vi "ReadandMedianSR830_ETH_copy2.vi"(0 "data storage rate (Hz)":u16(ring)=7 items=[".0625 ", "0.125 ", "0.250 ", "0.500 ", "1 ", "2 ", "4", "8 ", "16 ", "32 ", "64 ", "128", "256", "512"], 1 "Lockin Address":string="0:8", 2 "Integration (ms)":u32=10000, 3 "Delay (ms)":u32=3000, 4 "Measure Mode\n(T =Signal)":bool=TRUE, 5 "error in":T1) -> (6 "signal (complex)":cdb, 7 "Frequency (Hz)":dbl, 8 "error out":T1)   [LabVIEW 2023]
uses:
  <vilib>/Analysis/NI_AALBase.lvlib
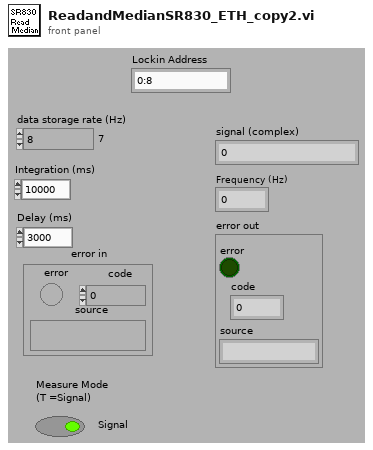
[diagram p1: front panel]
types:
  T1 = cluster{"error":bool, "code":i32, "source":string}
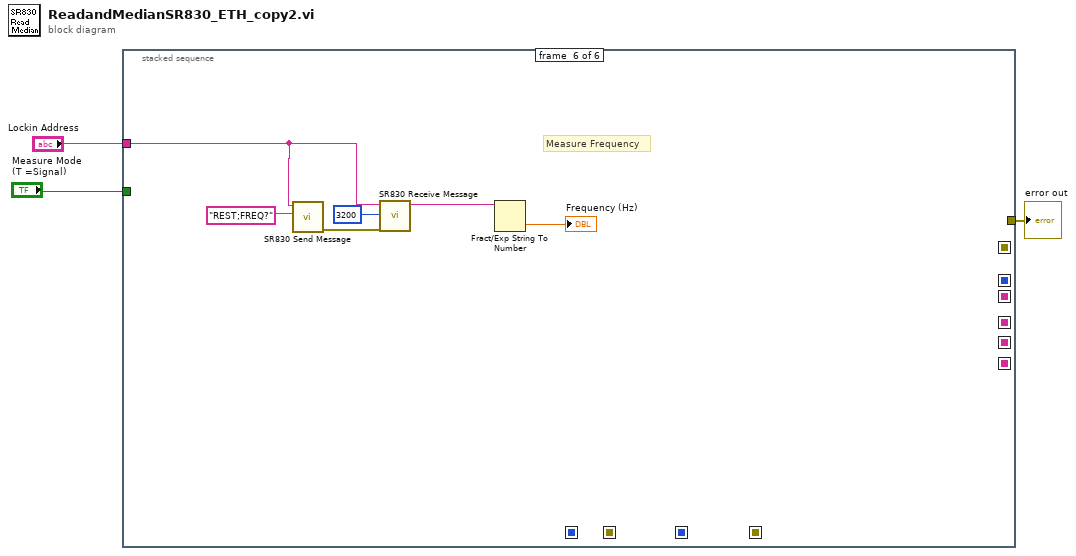
[diagram p0: block diagram]
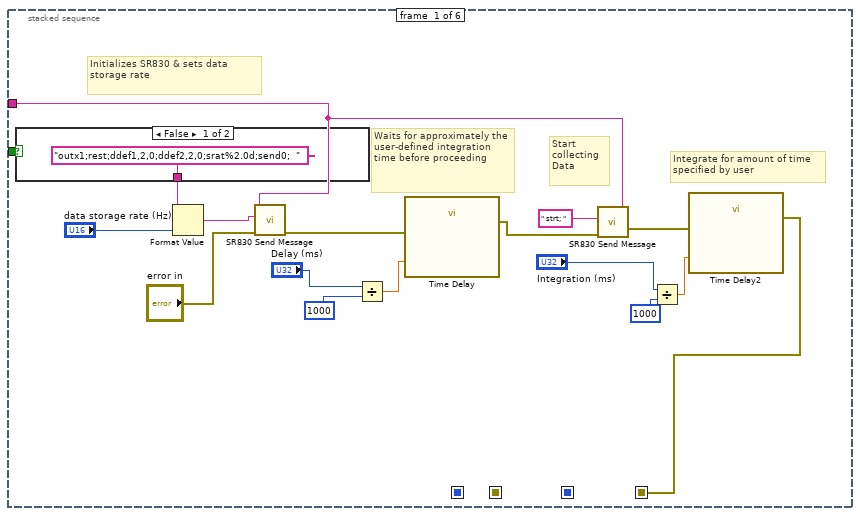
[diagram p2: hidden frame]
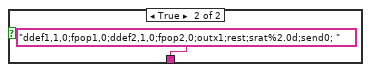
[diagram p3: hidden frame]
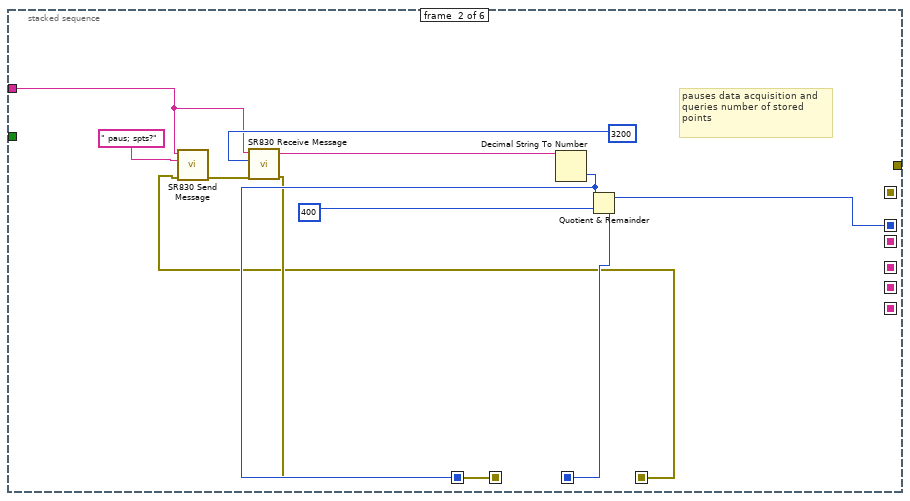
[diagram p4: hidden frame]
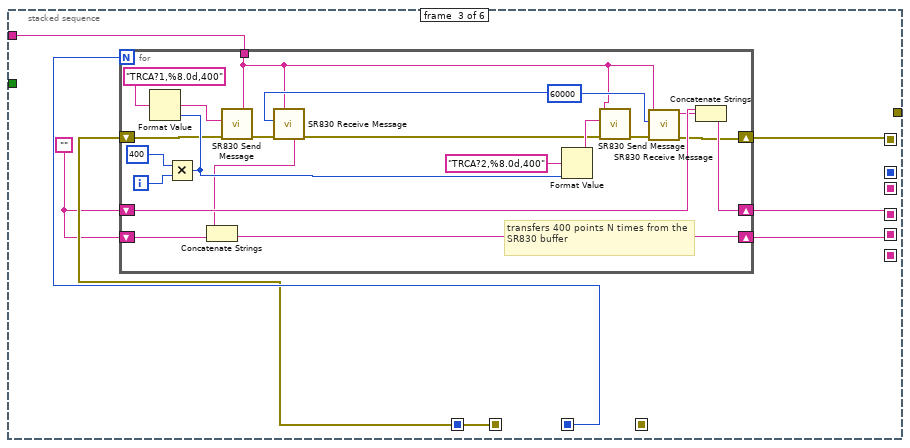
[diagram p5: hidden frame]
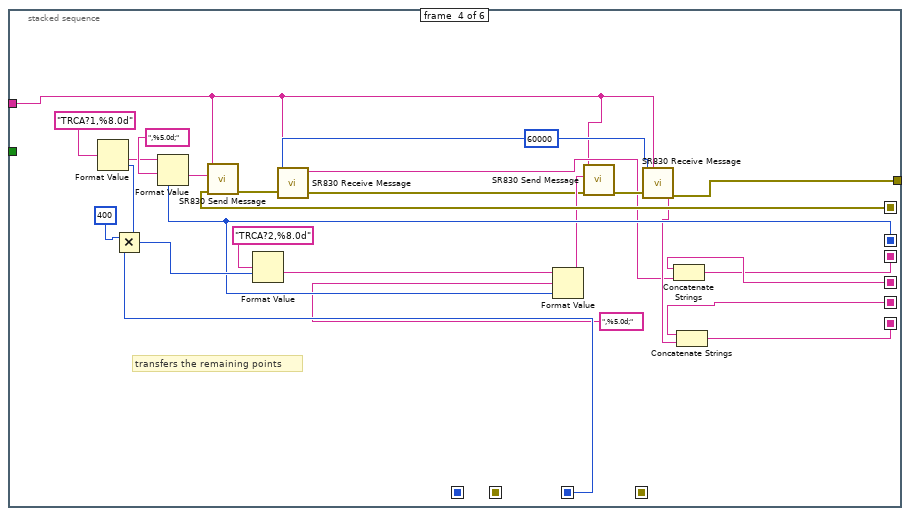
[diagram p6: hidden frame]
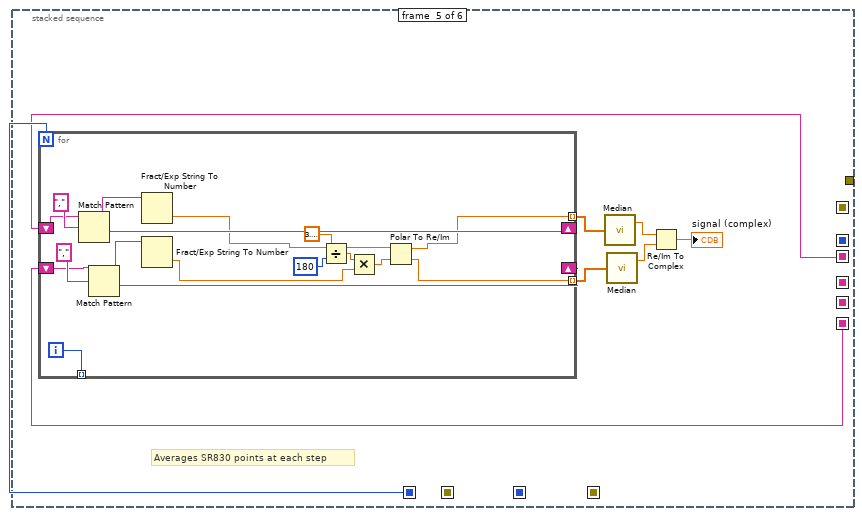
[diagram p7: hidden frame]
diagram:
  n1 = stacked-sequence {
    seq-local: [_ w32 _ _ _ _] -> [_ _ _ w82 _ _]
    seq-local: [_ w31 _ _ _ _] -> [_ _ w40 w84 _ _]
    seq-local: [_ w25 _ _ _ _] -> [_ _ w39 _ _ _]
    seq-local: [_ _ w37 _ _ _] -> [_ _ _ w79 _ _]
    seq-local: [_ _ w36 _ _ _] -> [_ _ _ w81 _ _]
    seq-local: [_ _ w35 _ _ _] -> [_ _ _ w80 _ _]
    seq-local: [_ w30 _ _ _ _] -> [_ _ _ _ w93 _]
    seq-local: [_ _ _ w64 _ _] -> [_ _ _ _ w91 _]
    seq-local: [_ _ _ w63 _ _] -> [_ _ _ _ w92 _]
    seq-local: [w17 _ _ _ _ _] -> [_ w24 _ _ _ _]
    tunnel: [_ _ _ w62 _ _] -> w3
    tunnel: "Lockin Address" -> [w5 w23 w34 w61 _ w116]
    tunnel: "Measure Mode\n(T =Signal)" -> [w4 _ _ _ _ _]
    frame #0 {
      # "Initializes SR830 & sets data storage rate"
      # "Integrate for amount of time\nspecified by user"
      # "Waits for approximately the user-defined integration time before proceeding"
      # "Start collecting Data"
      n2 = case shown="False" w4 {
        tunnel: ["outx1;rest;ddef1,2,0;ddef2,2,0;srat%2.0d;send0;  " "ddef1,1,0;fpop1,0;ddef2,1,0;fpop2,0;outx1;rest;srat%2.0d;send0; "] -> w15
        frame False {
        }
        frame True {
        }
      }
      n3 = Format Value(format string=w15, value (0)="data storage rate (Hz)") -> (output string=w13:string)  [unwired: 1 in]
      n4 = call "SR830 Send Message.vi"("address string"=w5, "write buffer"=w13, "error in"="error in") -> ("error out"=w16:T1)  [unwired: 4 in, 2 out]
      n5 = Divide(x="Delay (ms)", y=1000) -> (x/y=w9:dbl)
      n6 = call "Time Delay"("error in (no error)"=w16, "Delay Time (s)"=w9) -> ("error out"=w19:errorcluster)  [unwired: 9 in]
      n7 = call "SR830 Send Message.vi"("address string"=w5, "write buffer"=" strt; ", "error in"=w19) -> ("error out"=w18:T1)  [unwired: 4 in, 2 out]
      n8 = Divide(x="Integration (ms)", y=1000) -> (x/y=w6:dbl)
      n9 = call "Time Delay2"("error in (no error)"=w18, "Delay Time (s)"=w6) -> ("error out"=w17:errorcluster)  [unwired: 9 in]
    }
    frame #1 {
      # "pauses data acquisition and queries number of stored points"
      n10 = call "SR830 Send Message.vi"("address string"=w23, "write buffer"=" paus; spts?", "error in"=w24) -> ("error out"=w28:T1)  [unwired: 4 in, 2 out]
      n11 = call "SR830 Receive Message.vi"("address string"=w23, "byte count"=3200, "error in"=w28) -> ("read buffer"=w26:string, "error out"=w25:T1)  [unwired: 4 in, 1 out]
      n12 = Decimal String To Number(string=w26) -> (number=w30:i32)  [unwired: 2 in, 1 out]
      n13 = Quotient & Remainder(x=w30, y=400) -> (x-y*floor(x/y)=w32:i32, floor(x/y)=w31:i32)
    }
    frame #2 {
      w38 = ""
      n14 = for {
        N: w40 -> [_]
        shift-right: [w46] -> w37
        shift-left: w39 -> [w53]
        shift-right: [w58] -> w35
        shift-left: w38 -> [w57]
        shift-right: [w54] -> w36
        shift-left: w38 -> [w55]
        tunnel: w34 -> [w41]
        i -> [w60]
        w47 = 60000
        # "transfers 400 points N times from the SR830 buffer"
        n15 = Multiply(x=400, y=w60) -> (x*y=w56:i32)
        n16 = Format Value(format string="TRCA?1,%8.0d,400", value (0)=w56) -> (output string=w51:string)  [unwired: 1 in]
        n17 = call "SR830 Send Message.vi"("address string"=w41, "write buffer"=w51, "error in"=w53) -> ("error out"=w52:T1)  [unwired: 4 in, 2 out]
        n18 = call "SR830 Receive Message.vi"("address string"=w41, "byte count"=w47, "error in"=w52) -> ("read buffer"=w50:string, "error out"=w48:T1)  [unwired: 4 in, 1 out]
        n19 = Concatenate Strings(w50, w57) -> (w58:string)
        n20 = Format Value(format string="TRCA?2,%8.0d,400", value (0)=w56) -> (output string=w49:string)  [unwired: 1 in]
        n21 = call "SR830 Send Message.vi"("address string"=w41, "write buffer"=w49, "error in"=w48) -> ("error out"=w45:T1)  [unwired: 4 in, 2 out]
        n22 = call "SR830 Receive Message.vi"("address string"=w41, "byte count"=w47, "error in"=w45) -> ("read buffer"=w44:string, "error out"=w46:T1)  [unwired: 4 in, 1 out]
        n23 = Concatenate Strings(w55, w44) -> (w54:string)
      }
    }
    frame #3 {
      w73 = 60000
      # "transfers the remaining points"
      n24 = Multiply(x=400, y=w84) -> (x*y=w83:i32)
      n25 = Format Value(format string="TRCA?1,%8.0d", value (0)=w83) -> (output string=w69:string)  [unwired: 1 in]
      n26 = Format Value(string ("")=w69, format string=",%5.0d;", value (0)=w82) -> (output string=w68:string)
      n27 = call "SR830 Send Message.vi"("address string"=w61, "write buffer"=w68, "error in"=w79) -> ("error out"=w75:T1)  [unwired: 4 in, 2 out]
      n28 = Format Value(format string="TRCA?2,%8.0d", value (0)=w83) -> (output string=w65:string)  [unwired: 1 in]
      n29 = call "SR830 Receive Message.vi"("address string"=w61, "byte count"=w73, "error in"=w75) -> ("read buffer"=w74:string, "error out"=w72:T1)  [unwired: 4 in, 1 out]
      n30 = Format Value(string ("")=w65, format string=",%5.0d;", value (0)=w82) -> (output string=w78:string)
      n31 = call "SR830 Send Message.vi"("address string"=w61, "write buffer"=w78, "error in"=w72) -> ("error out"=w77:T1)  [unwired: 4 in, 2 out]
      n32 = call "SR830 Receive Message.vi"("address string"=w61, "byte count"=w73, "error in"=w77) -> ("read buffer"=w76:string, "error out"=w62:T1)  [unwired: 4 in, 1 out]
      n33 = Concatenate Strings(w81, w74) -> (w64:string)
      n34 = Concatenate Strings(w80, w76) -> (w63:string)
    }
    frame #4 {
      # "Averages SR830 points at each step"
      n35 = for {
        N: w93 -> [_]
        shift-right: [w106] -> _
        shift-left: w91 -> [w105]
        shift-right: [w104] -> _
        shift-left: w92 -> [w103]
        tunnel: [w102] -> _ mode=indexing
        tunnel: [w99] -> w89 mode=indexing
        tunnel: [w98] -> w88 mode=indexing
        i -> [w102]
        n36 = Match Pattern(string=w105, regular expression=",") -> (before substring=w109:string, after substring=w106:string)  [unwired: 1 in, 2 out]
        n37 = Match Pattern(string=w103, regular expression=",") -> (before substring=w108:string, after substring=w104:string)  [unwired: 1 in, 2 out]
        n38 = Fract/Exp String To Number(string=w109) -> (number=w100:dbl)  [unwired: 3 in, 1 out]
        n39 = Fract/Exp String To Number(string=w108) -> (number=w101:dbl)  [unwired: 3 in, 1 out]
        n40 = Divide(x=3.141592653589793, y=180) -> (x/y=w95:dbl)
        n41 = Multiply(x=w95, y=w101) -> (x*y=w94:dbl)
        n42 = Polar To Re/Im(2:w94, 3:w100) -> (0:w98:dbl, 1:w99:dbl)
      }
      n43 = call <vilib>:"Median.vi"("X"=w89) -> ("median"=w86:dbl)  [unwired: 1 out]
      n44 = call <vilib>:"Median.vi"("X"=w88) -> ("median"=w87:dbl)  [unwired: 1 out]
      n45 = Re/Im To Complex(1:w87, 2:w86) -> (0:→"signal (complex)":cdb)
    }
    frame #5 {
      # "Measure Frequency"
      n46 = call "SR830 Send Message.vi"("address string"=w116, "write buffer"="REST;FREQ?") -> ("error out"=w114:T1)  [unwired: 5 in, 2 out]
      n47 = call "SR830 Receive Message.vi"("address string"=w116, "byte count"=3200, "error in"=w114) -> ("read buffer"=w113:string)  [unwired: 4 in, 2 out]
      n48 = Fract/Exp String To Number(string=w113) -> (number=→"Frequency (Hz)":dbl)  [unwired: 3 in, 1 out]
    }
  }
  "error out" <- w3
